vi "Device Outputs Write.vi"(8 "error in (no error)":errorcluster, 10 "Device Outputs":dbl[](array[numeric]), 11 "DCM-NIVS-RT in":refnum<class "DCM-NIVS-RT.lvclass">) -> (0 "error out":errorcluster, 3 "DCM-NIVS-RT out":refnum<class "DCM-NIVS-RT.lvclass">)   [LabVIEW 2016, in "DCM Engine.lvlib" / "DCM-NIVS-RT.lvclass"]
uses:
  DCM-NIVS-RT.lvclass
  DCM-NIVS-RT.lvclass/DCM-NIVS-RT.ctl
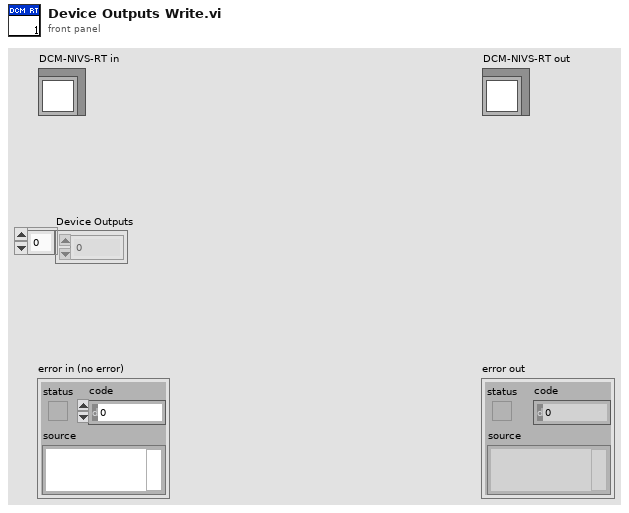
[diagram p1: front panel]
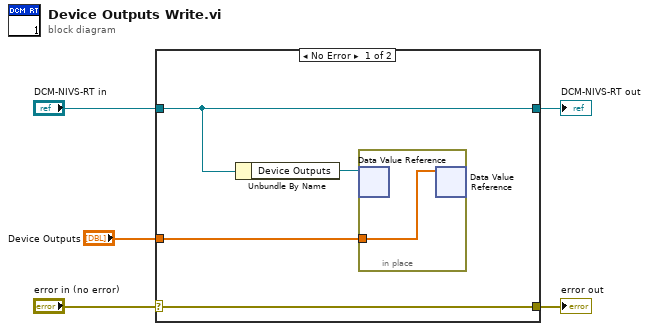
[diagram p0: block diagram]
diagram:
  n1 = case shown="No Error" "error in (no error)" {
    selector: "error in (no error)" -> [w9 w12]
    tunnel: [w9 w12] -> w4
    tunnel: [w8 w11] -> w2
    tunnel: "DCM-NIVS-RT in" -> [w8 w11]
    tunnel: "Device Outputs" -> [w6 _]
    frame No Error {
      n2 = Unbundle By Name(w8) -> ("Device Outputs"=w7:refnum<data-value>)
      n3 = in-place {
        in-place-border: w6 -> [w10]
        n4 = in-place-dvr #1(w7) -> ()  [unwired: 2 out]
        n5 = in-place-dvr #1(w10) -> ()  [unwired: 2 out]
      }
    }
    frame Error {
    }
  }
  "error out" <- w4
  "DCM-NIVS-RT out" <- w2
